vi "Actor Core.vi"(8 "error in":errorcluster, 11 "Nested in":refnum<class "UI Actor.lvclass">) -> (0 "error out":errorcluster, 3 "Actor out":refnum<class "Actor.lvclass">)   [LabVIEW 2020, in "UI Actor.lvlib" / "UI Actor.lvclass"]
doc: "(<B>Filename</B>: Actor Framework.lvlib:Actor.lvclass:Actor Core.vi)\n\nReceives messages to the actor, reacts to them, and initiates any error handling that may shut the actor down.\n\nDescendant classes may override this VI to append parallel tasks for the actor to complete while it handles messages. Overrides use the Call Parent Method node."
uses:
  UI Actor.lvclass
  C:/Program Files/National Instruments/LabVIEW 2020/vi.lib/ActorFramework/Actor/Actor.lvclass
  <vilib>/ActorFramework/Actor/Actor.lvclass
  UI Actor.lvclass/UI Actor.ctl
  <vilib>/ActorFramework/Actor/Actor.lvclass/Actor.ctl
  <vilib>/ActorFramework/Message Enqueuer/Message Enqueuer.lvclass/Message Enqueuer.ctl
  Write Sub Panel Prod.vi
  Write Sub Panel Monedas.vi
  Write Sub Panel Mensajes.vi
  <vilib>/ActorFramework/Message Enqueuer/Init from Existing Queue.vi
  <vilib>/ActorFramework/Message Enqueuer/Enqueue.vi
  <vilib>/ActorFramework/Stop Msg/Stop Msg.lvclass
  C:/Program Files/National Instruments/LabVIEW 2020/vi.lib/ActorFramework/Message/Message.lvclass
  <vilib>/ActorFramework/Message Priority Queue/Priority Enqueue.vi
  <vilib>/ActorFramework/Message Enqueuer/Message Enqueuer.lvclass
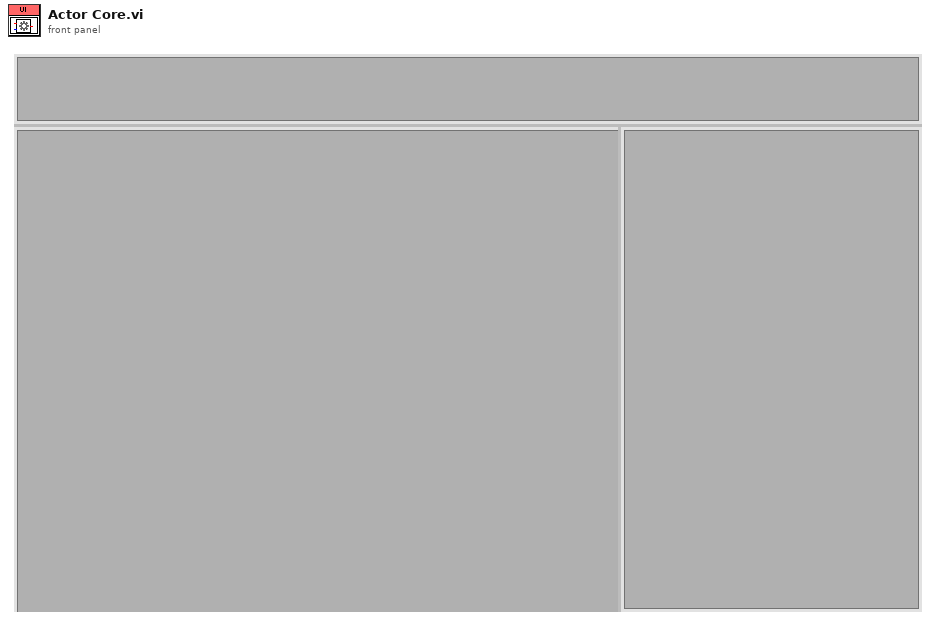
[diagram p1: front panel]
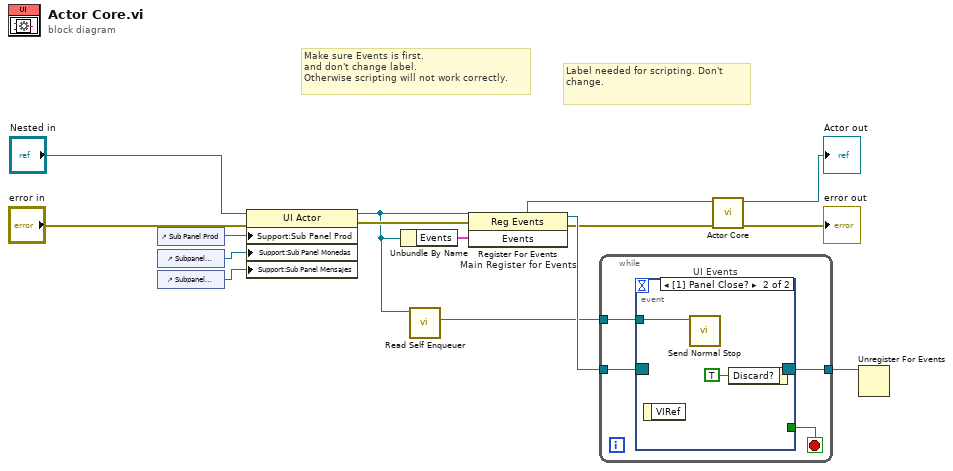
[diagram p0: block diagram]
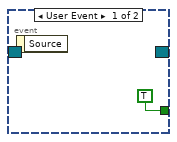
[diagram p2: hidden frame]
diagram:
  # "Label needed for scripting. Don't change."
  # "Make sure Events is first.\nand don't change label.\nOtherwise scripting will not work correctly."
  n1 = control-ref of="Sub Panel Prod"() -> (w3:refnum<vi>)
  n2 = control-ref of="Subpanel monedas"() -> (w2:refnum<vi>)
  n3 = control-ref of="Subpanel mensajes"() -> (w1:refnum<vi>)
  n4 = property class="UI Actor"(reference="Nested in", error in="error in", "Support:Sub Panel Prod"=w3, "Support:Sub Panel Monedas"=w2, "Support:Sub Panel Mensajes"=w1) -> (reference out=w4:refnum<class "UI Actor.lvclass">, error out=w5:errorcluster)
  n5 = Unbundle By Name(w4) -> ("Events"=w11:cluster{"Stop":refnum<user-event>})
  n6 = call <vilib>:"Read Self Enqueuer.vi"("Actor"=w4) -> ("Self Enqueuer"=w8:refnum<class "Message Enqueuer.lvclass">)  [unwired: 10 in]
  n7 = register-events "Main Register for Events"(error in=w5, w11) -> (reference out=w12:refnum<event-registration>, error out=w7:errorcluster)  [unwired: 1 in]
  n8 = while {
    tunnel: w12 -> [w18]
    tunnel: [w16] -> w10
    tunnel: w8 -> [w15]
    stop <- w17 stop-if-true
    n9 = event "UI Events" shown="[1] Panel Close?" {
      selector: w18 -> [_ _]
      dyn-events: [_ _] -> w16
      timeout: _ -> [_ _]
      tunnel: [TRUE _] -> w17
      tunnel: w15 -> [_ w20]
      event User Event {
        n10 = event-data() -> ()  [unwired: 1 in, 1 out]
      }
      event Panel Close? {
        n11 = event-data() -> ()  [unwired: 1 in, 1 out]
        n12 = call <vilib>:"Send Normal Stop.vi"("Message Enqueuer"=w20) -> ()  [unwired: 10 in, 1 out]
        n13 = event-data("Discard?"=TRUE) -> ()  [unwired: 1 in, 1 out]
      }
    }
  }
  n14 = call-parent "Actor Core.vi"("error in"=w7, "Actor in"=w4) -> ("error out"=→"error out":errorcluster, "Actor out"=→"Actor out":refnum<class "Actor.lvclass">)  [unwired: 8 in]
  n15 = Unregister For Events(event registration refnum=w10) -> ()  [unwired: 1 in, 1 out]
